vi "Actividad2.2.vi"() -> ()   [LabVIEW 2026]
panel:
  in  "stop":bool
  out "Tank 2":dbl(slide) scale=0.0..10.0
  out "Valvula Final":bool
  out "M":bool
  out "V1":bool
  in  "D_alto":bool
  in  "D_bajo":bool
  out "V2":bool
  in  "SP2":bool
  in  "SP1":bool
  out "VB":bool
  out "VA":bool
  out "Tank 1":dbl(slide) scale=0.0..10.0
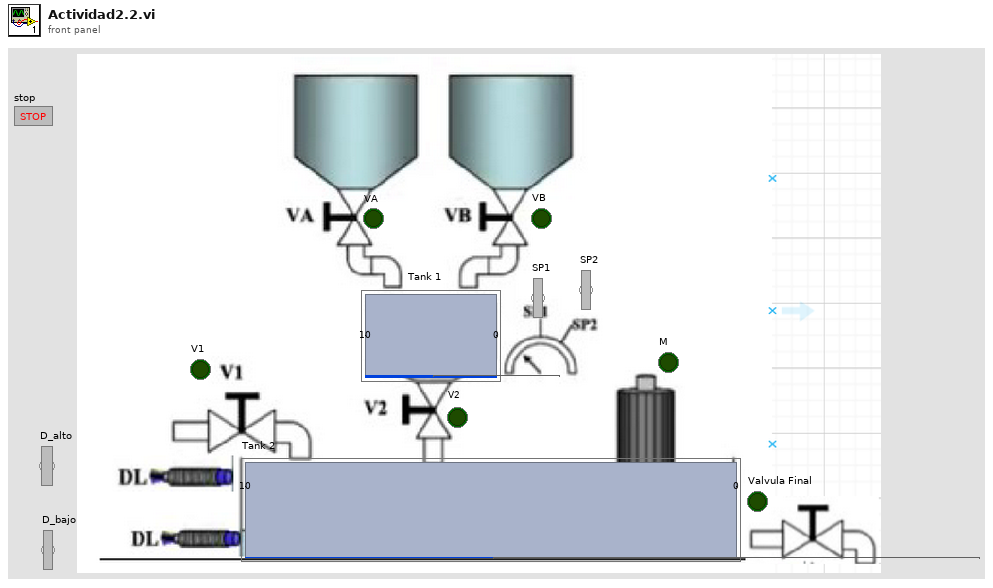
[diagram p1: front panel]
types:
  T1 = enum16{"Estado0", "Estado1", "Estado2", "Estado3", "Estado4", "Estado5", "Estado6", "Estado7", ""}
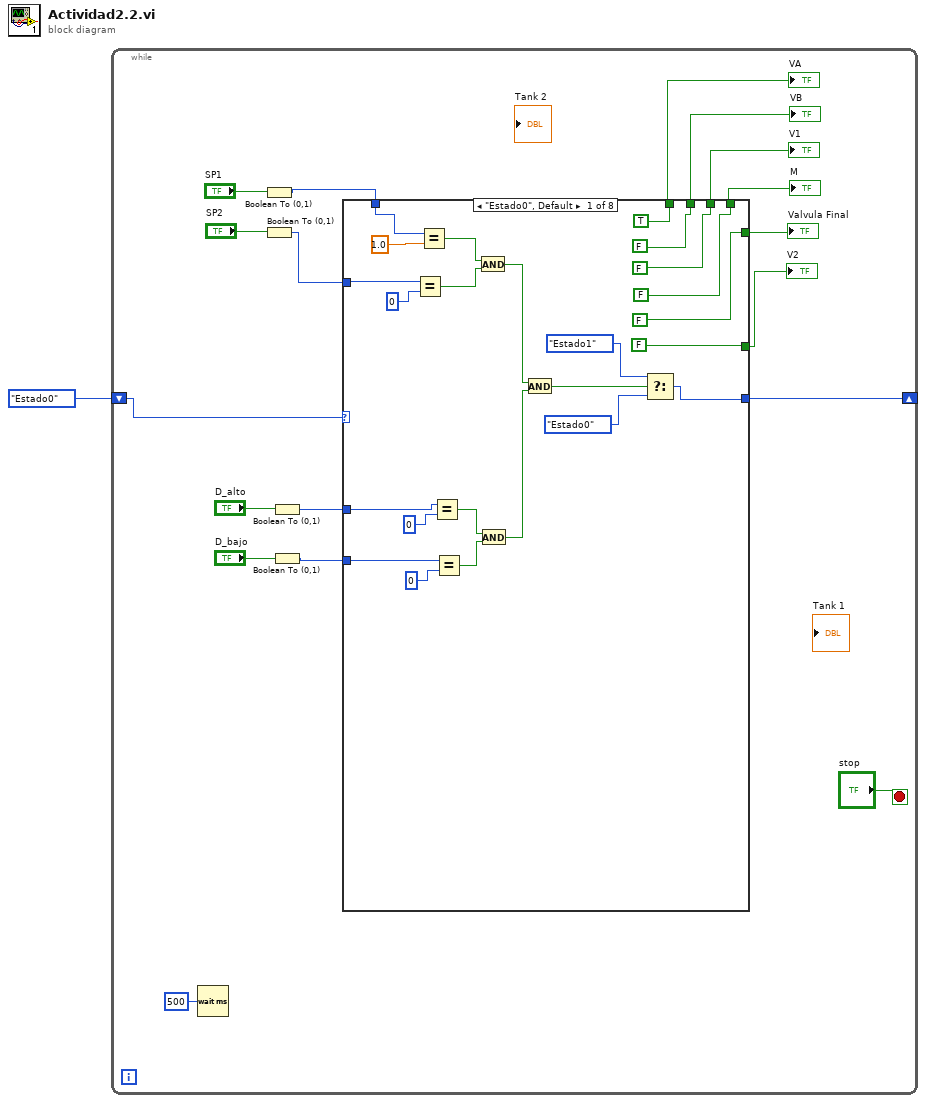
[diagram p0: block diagram]
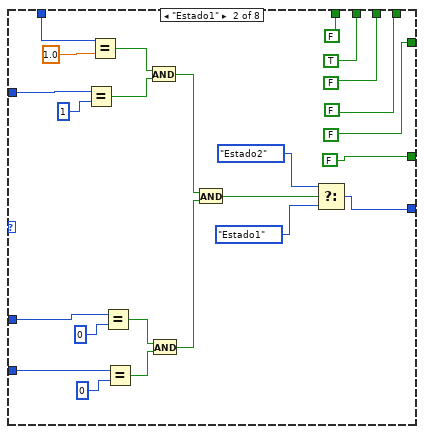
[diagram p2: hidden frame]
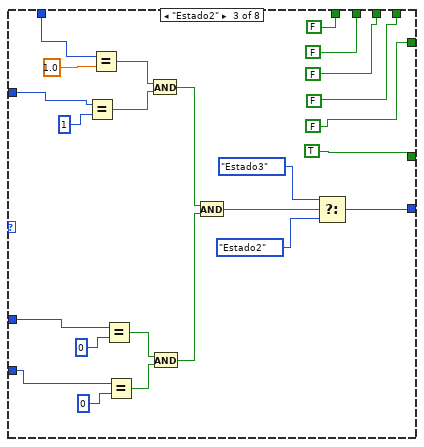
[diagram p3: hidden frame]
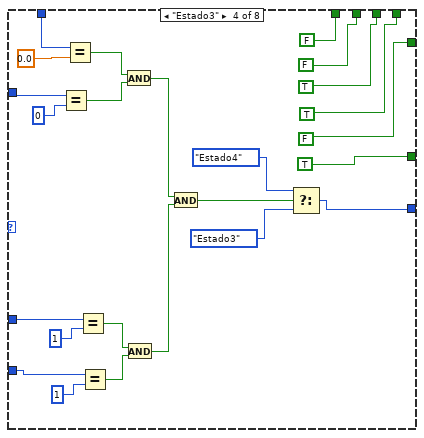
[diagram p4: hidden frame]
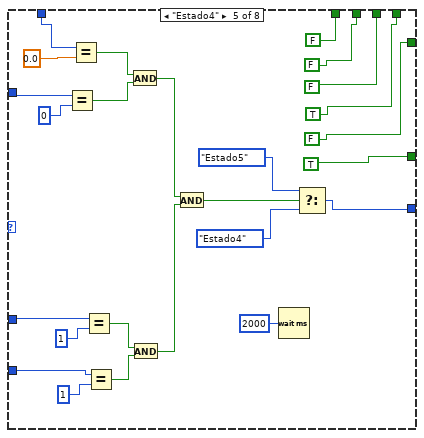
[diagram p5: hidden frame]
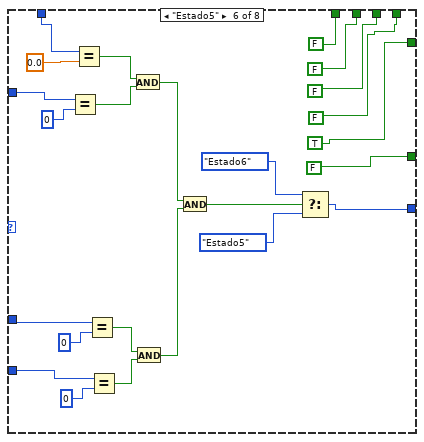
[diagram p6: hidden frame]
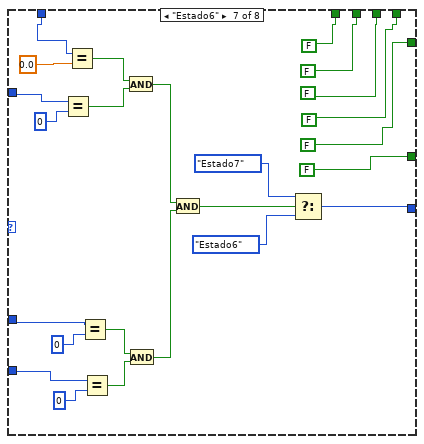
[diagram p7: hidden frame]
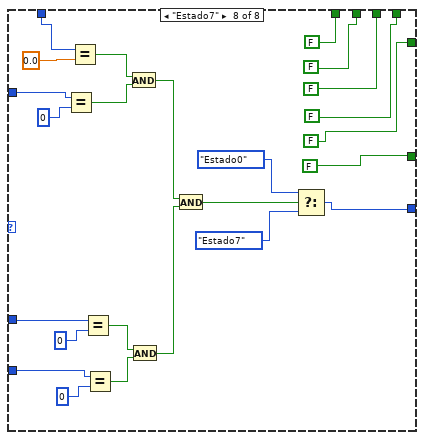
[diagram p8: hidden frame]
diagram:
  n1 = while {
    shift-right: [w5] -> _
    shift-left: T1."Estado0" -> [w18]
    stop <- "stop" stop-if-true
    n2 = Wait (ms)(milliseconds to wait=u32 500) -> ()  [unwired: 1 out]
    n3 = Boolean To (0,1)(Boolean="SP1") -> (0, 1=w9:i16)
    n4 = Boolean To (0,1)(Boolean="SP2") -> (0, 1=w8:i16)
    n5 = Boolean To (0,1)(Boolean="D_alto") -> (0, 1=w7:i16)
    n6 = Boolean To (0,1)(Boolean="D_bajo") -> (0, 1=w6:i16)
    n7 = case shown="\"Estado0\", Default" w18 {
      tunnel: [TRUE FALSE FALSE FALSE FALSE FALSE FALSE FALSE] -> w17
      tunnel: [FALSE TRUE FALSE FALSE FALSE FALSE FALSE FALSE] -> w16
      tunnel: [FALSE FALSE FALSE TRUE FALSE FALSE FALSE FALSE] -> w15
      tunnel: [FALSE FALSE FALSE TRUE TRUE FALSE FALSE FALSE] -> w14
      tunnel: [FALSE FALSE FALSE FALSE FALSE TRUE FALSE FALSE] -> w13
      tunnel: [FALSE FALSE TRUE TRUE TRUE FALSE FALSE FALSE] -> w12
      tunnel: w9 -> [w30 w60 w77 w102 w127 w151 w175 w192]
      tunnel: w8 -> [w29 w59 w76 w101 w117 w150 w174 w191]
      tunnel: w7 -> [w28 w55 w75 w94 w126 w149 w173 w190]
      tunnel: w6 -> [w27 w54 w74 w93 w125 w148 w172 w189]
      tunnel: [w20 w44 w78 w92 w118 w141 w165 w193] -> w5
      frame "Estado0", Default {
        n8 = Equal?(x=w29, y=i16 0) -> (x = y?=w38:bool)
        n9 = Equal?(x=w30, y=1.0) -> (x = y?=w39:bool)
        n10 = Equal?(x=w28, y=i16 0) -> (x = y?=w37:bool)
        n11 = Equal?(x=w27, y=i16 0) -> (x = y?=w36:bool)
        n12 = And(x=w39, y=w38) -> (x .and. y?=w35:bool)
        n13 = And(x=w37, y=w36) -> (x .and. y?=w34:bool)
        n14 = And(x=w35, y=w34) -> (x .and. y?=w33:bool)
        n15 = Select(t=T1."Estado1", s=w33, f=T1."Estado0") -> (s? t:f=w20:T1)
      }
      frame "Estado1" {
        n16 = Equal?(x=w59, y=i16 1) -> (x = y?=w52:bool)
        n17 = Equal?(x=w60, y=1.0) -> (x = y?=w53:bool)
        n18 = Equal?(x=w55, y=i16 0) -> (x = y?=w51:bool)
        n19 = Equal?(x=w54, y=i16 0) -> (x = y?=w50:bool)
        n20 = And(x=w53, y=w52) -> (x .and. y?=w49:bool)
        n21 = And(x=w51, y=w50) -> (x .and. y?=w48:bool)
        n22 = And(x=w49, y=w48) -> (x .and. y?=w47:bool)
        n23 = Select(t=T1."Estado2", s=w47, f=T1."Estado1") -> (s? t:f=w44:T1)
      }
      frame "Estado2" {
        n24 = Equal?(x=w76, y=i16 1) -> (x = y?=w86:bool)
        n25 = Equal?(x=w77, y=1.0) -> (x = y?=w87:bool)
        n26 = Equal?(x=w75, y=i16 0) -> (x = y?=w85:bool)
        n27 = Equal?(x=w74, y=i16 0) -> (x = y?=w84:bool)
        n28 = And(x=w87, y=w86) -> (x .and. y?=w83:bool)
        n29 = And(x=w85, y=w84) -> (x .and. y?=w82:bool)
        n30 = And(x=w83, y=w82) -> (x .and. y?=w81:bool)
        n31 = Select(t=T1."Estado3", s=w81, f=T1."Estado2") -> (s? t:f=w78:T1)
      }
      frame "Estado3" {
        n32 = Equal?(x=w101, y=i16 0) -> (x = y?=w110:bool)
        n33 = Equal?(x=w102, y=0.0) -> (x = y?=w111:bool)
        n34 = Equal?(x=w94, y=i16 1) -> (x = y?=w109:bool)
        n35 = Equal?(x=w93, y=i16 1) -> (x = y?=w108:bool)
        n36 = And(x=w111, y=w110) -> (x .and. y?=w107:bool)
        n37 = And(x=w109, y=w108) -> (x .and. y?=w106:bool)
        n38 = And(x=w107, y=w106) -> (x .and. y?=w105:bool)
        n39 = Select(t=T1."Estado4", s=w105, f=T1."Estado3") -> (s? t:f=w92:T1)
      }
      frame "Estado4" {
        n40 = Equal?(x=w117, y=i16 0) -> (x = y?=w135:bool)
        n41 = Equal?(x=w127, y=0.0) -> (x = y?=w136:bool)
        n42 = Equal?(x=w126, y=i16 1) -> (x = y?=w134:bool)
        n43 = Equal?(x=w125, y=i16 1) -> (x = y?=w133:bool)
        n44 = And(x=w136, y=w135) -> (x .and. y?=w132:bool)
        n45 = And(x=w134, y=w133) -> (x .and. y?=w131:bool)
        n46 = And(x=w132, y=w131) -> (x .and. y?=w130:bool)
        n47 = Wait (ms)(milliseconds to wait=u32 2000) -> ()  [unwired: 1 out]
        n48 = Select(t=T1."Estado5", s=w130, f=T1."Estado4") -> (s? t:f=w118:T1)
      }
      frame "Estado5" {
        n49 = Equal?(x=w150, y=i16 0) -> (x = y?=w159:bool)
        n50 = Equal?(x=w151, y=0.0) -> (x = y?=w160:bool)
        n51 = Equal?(x=w149, y=i16 0) -> (x = y?=w158:bool)
        n52 = Equal?(x=w148, y=i16 0) -> (x = y?=w157:bool)
        n53 = And(x=w160, y=w159) -> (x .and. y?=w156:bool)
        n54 = And(x=w158, y=w157) -> (x .and. y?=w155:bool)
        n55 = And(x=w156, y=w155) -> (x .and. y?=w154:bool)
        n56 = Select(t=T1."Estado6", s=w154, f=T1."Estado5") -> (s? t:f=w141:T1)
      }
      frame "Estado6" {
        n57 = Equal?(x=w174, y=i16 0) -> (x = y?=w183:bool)
        n58 = Equal?(x=w175, y=0.0) -> (x = y?=w184:bool)
        n59 = Equal?(x=w173, y=i16 0) -> (x = y?=w182:bool)
        n60 = Equal?(x=w172, y=i16 0) -> (x = y?=w181:bool)
        n61 = And(x=w184, y=w183) -> (x .and. y?=w180:bool)
        n62 = And(x=w182, y=w181) -> (x .and. y?=w179:bool)
        n63 = And(x=w180, y=w179) -> (x .and. y?=w178:bool)
        n64 = Select(t=T1."Estado7", s=w178, f=T1."Estado6") -> (s? t:f=w165:T1)
      }
      frame "Estado7" {
        n65 = Equal?(x=w191, y=i16 0) -> (x = y?=w207:bool)
        n66 = Equal?(x=w192, y=0.0) -> (x = y?=w208:bool)
        n67 = Equal?(x=w190, y=i16 0) -> (x = y?=w206:bool)
        n68 = Equal?(x=w189, y=i16 0) -> (x = y?=w205:bool)
        n69 = And(x=w208, y=w207) -> (x .and. y?=w204:bool)
        n70 = And(x=w206, y=w205) -> (x .and. y?=w203:bool)
        n71 = And(x=w204, y=w203) -> (x .and. y?=w202:bool)
        n72 = Select(t=T1."Estado0", s=w202, f=T1."Estado7") -> (s? t:f=w193:T1)
      }
    }
    "VA" <- w17
    "VB" <- w16
    "V2" <- w12
    "V1" <- w15
    "M" <- w14
    "Valvula Final" <- w13
  }
